vi "Interpolate Signal (Number).vi"(2 "desired # of points":i32, 3 "Array":dbl[](array[numeric]) format="%.2f") -> (1 "Resampled Array":dbl[](array[numeric]))   [LabVIEW 2019]
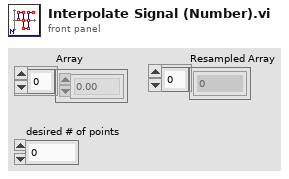
[diagram p1: front panel]
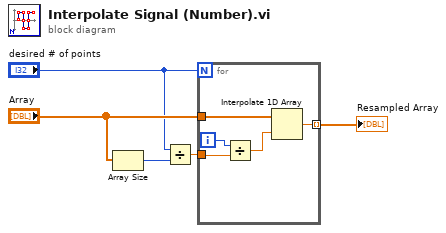
[diagram p0: block diagram]
diagram:
  n1 = Array Size(array="Array") -> (size(s)=w2:i32)
  n2 = Divide(x="desired # of points", y=w2) -> (x/y=w3:dbl)
  n3 = for {
    N: "desired # of points" -> [_]
    tunnel: w3 -> [w7]
    tunnel: "Array" -> [w9]
    tunnel: [w8] -> w5 mode=indexing
    i -> [w6]
    n4 = Divide(x=w6, y=w7) -> (x/y=w10:dbl)
    n5 = Interpolate 1D Array(1:w10, 2:w9) -> (0:w8:dbl)
  }
  "Resampled Array" <- w5
